vi "Write Shift.vi"(8 "error in (no error)":errorcluster, 10 "Shift":bool, 11 "KeyDown in":refnum<class "KeyDown.lvclass">) -> (0 "error out":errorcluster, 3 "KeyDown out":refnum<class "KeyDown.lvclass">)   [LabVIEW 2016, in "DataGrid.lvlib" / "KeyDown.lvclass"]
uses:
  <userlib>/LabVIEWdotNetDataGrid/source/Events/KeyDown/KeyDown.lvclass
  <userlib>/LabVIEWdotNetDataGrid/source/Events/KeyDown/KeyDown.lvclass/KeyDown.ctl
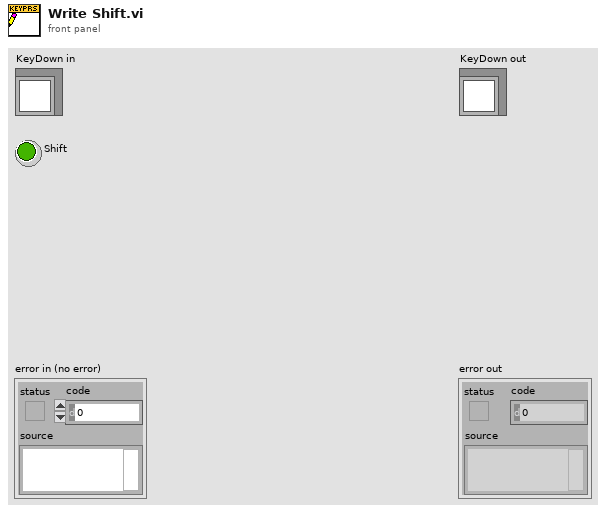
[diagram p1: front panel]
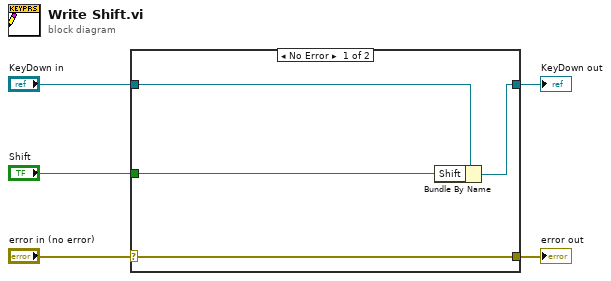
[diagram p0: block diagram]
diagram:
  n1 = case shown="No Error" "error in (no error)" {
    selector: "error in (no error)" -> [w9 w10]
    tunnel: [w9 w10] -> w4
    tunnel: [w7 w11] -> w2
    tunnel: "KeyDown in" -> [w8 w11]
    tunnel: "Shift" -> [w6 _]
    frame No Error {
      n2 = Bundle By Name(cluster=w8, "Shift"=w6) -> (w7:refnum<class "KeyDown.lvclass">)
    }
    frame Error {
    }
  }
  "error out" <- w4
  "KeyDown out" <- w2
